vi "Steppers_and_Scanners_control_5_24.vi"(1 "ANC300 address":refnum<visa-resource-name>="COM8") -> (18 "Serial":string="ANC300B-C-2133-4009033")   [LabVIEW 2022 SP3]
panel:
  in  "wait time (ms)":u32=1
  out "2: Voltage Reading":dbl format="%#_13g"
  out "1: Voltage Reading":dbl format="%#_13g"
  in  "Set/Read":bool=TRUE
  in  "Stepper 4":bool
  in  "4: ms to wait":u32=1
  in  "4: number of steps":i32=1
  in  "4: stepping direction":bool=TRUE
  in  "4: AC Voltage":dbl=1.0 min=0.0 format="%.1g"
  in  "4: AC frequency":dbl=10.0 min=0.0 format="%.1f"
  in  "Stepper 3":bool
  in  "3: ms to wait":u32=1
  in  "3: number of steps":i32=1
  in  "3: stepping direction":bool=TRUE
  in  "3: AC Voltage":dbl=1.0 min=0.0 format="%.1g"
  in  "3: AC frequency":dbl=10.0 min=0.0 format="%.1f"
  in  "2: ms to wait":u32=1
  in  "2: Offset Voltage":dbl min=0.0 format="%.1g"
  in  "1: ms to wait":u32=1
  in  "1: Offset Voltage":dbl min=0.0 format="%.1g"
  # "Scanner 1"
  # "Scanner 2"
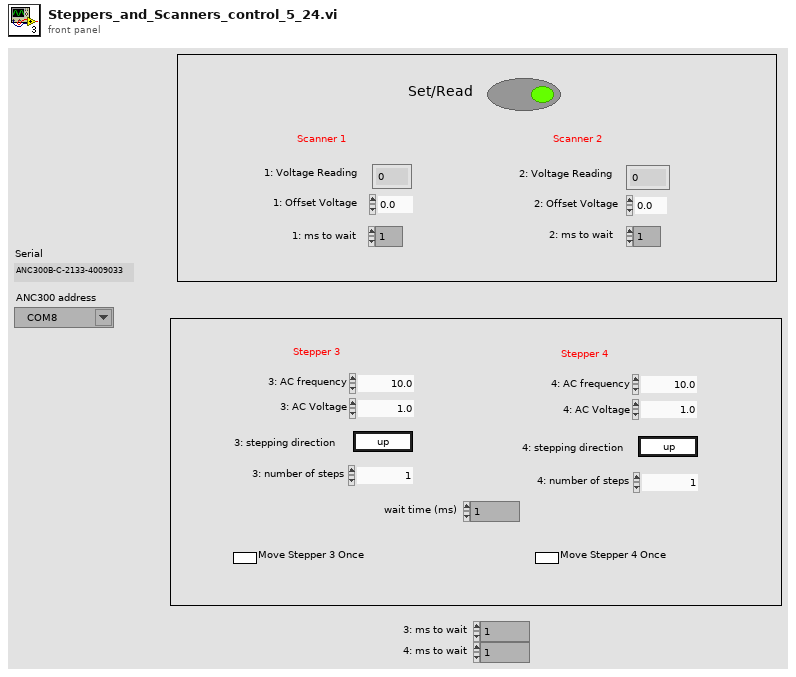
[diagram p1: front panel]
types:
  T1 = cluster{"error ":bool, "error number":i32, "error code":string}
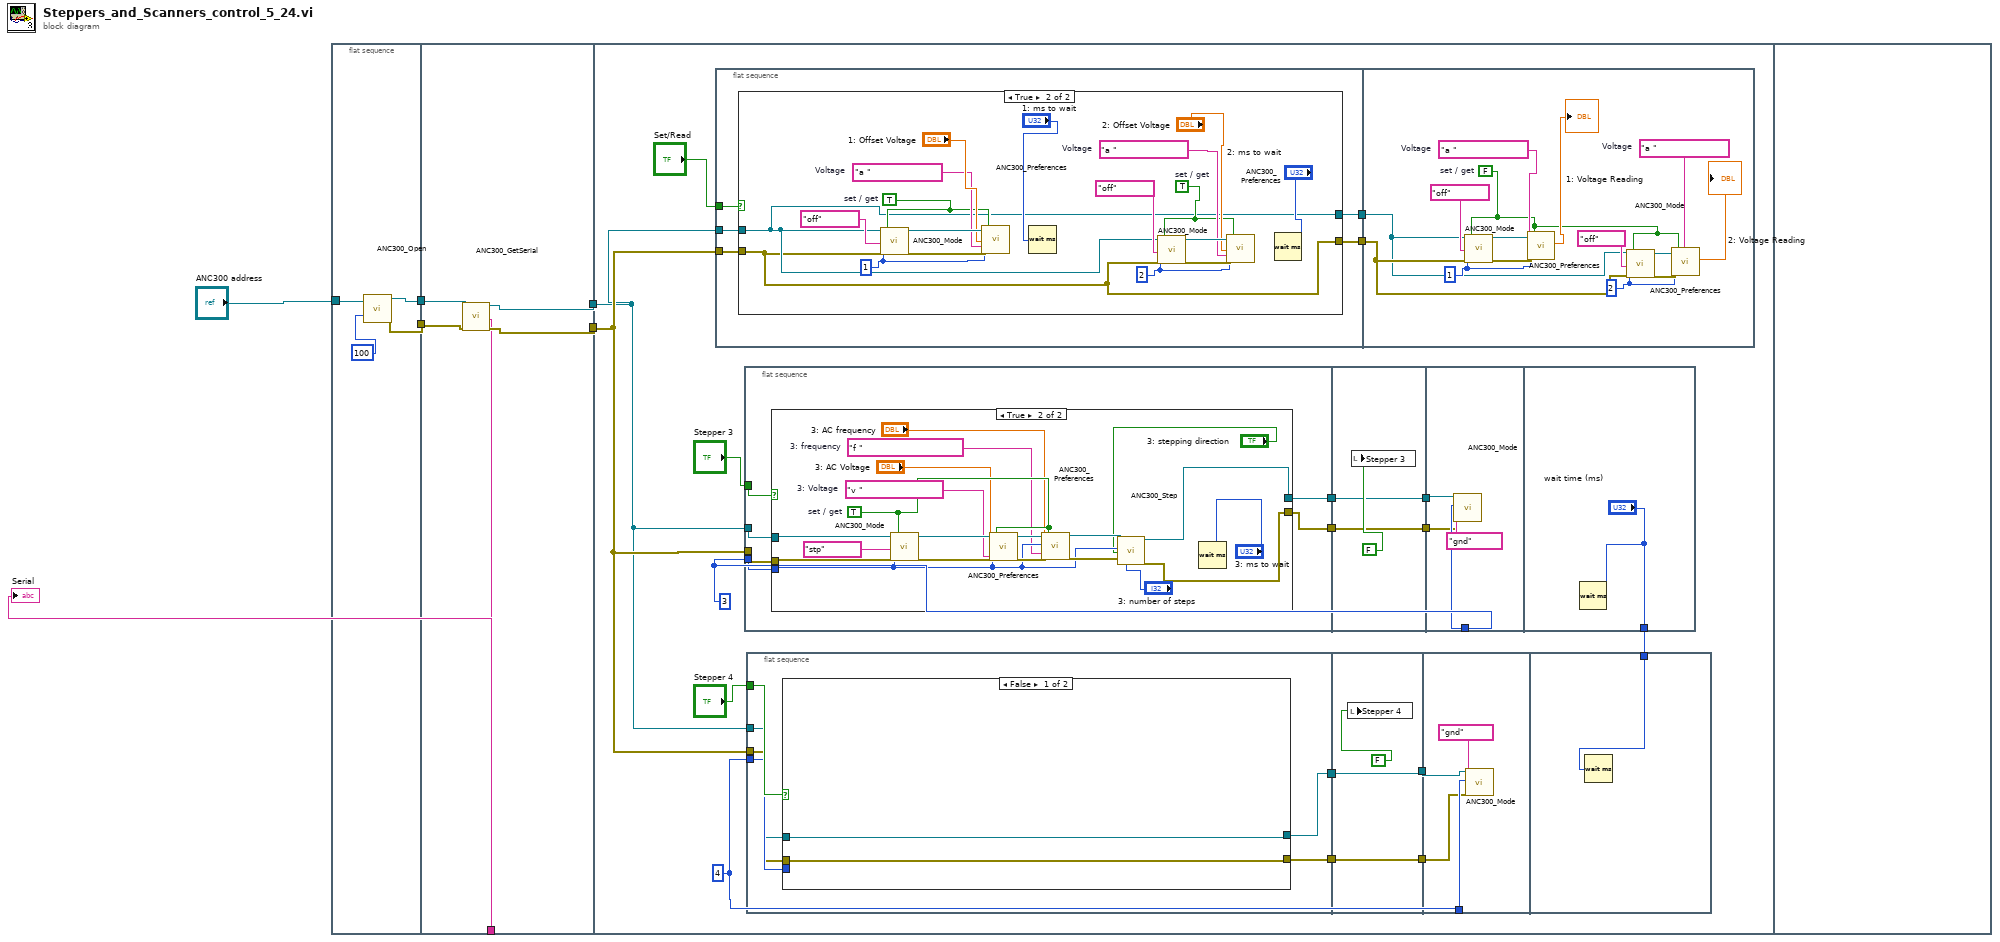
[diagram p0: block diagram]
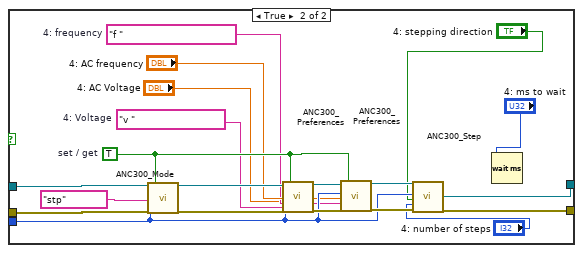
[diagram p4: hidden frame]
diagram:
  n1 = flat-sequence {
    tunnel: "ANC300 address" -> [w9]
    tunnel: [w10] -> w6
    tunnel: [w8] -> w5
    tunnel: w6 -> [w15]
    tunnel: w5 -> [w14]
    tunnel: [w13] -> w4
    tunnel: [w12] -> w3
    tunnel: [w11] -> w2
    tunnel: w4 -> [w30]
    tunnel: w3 -> [w31]
    frame #0 {
      n2 = call "ANC300_Open.vi"("ANC300 Communication Port In"=w9, "milliseconds to wait"=u32 100 ("millisecond timer value")) -> ("ANC300 Communication Port Out"=w10:refnum<visa-resource-name>, "error out"=w8:T1)  [unwired: 13 in, 3 out]
    }
    frame #1 {
      n3 = call "ANC300_GetSerial.vi"("ANC300 Communication Port In"=w15, "error in"=w14) -> ("ANC300 Communication Port Out"=w13:refnum<visa-resource-name>, "Serial"=w11:string, "error out"=w12:T1)  [unwired: 10 in, 5 out]
    }
    frame #2 {
      w29 = 3
      w32 = 4
      n4 = flat-sequence {
        tunnel: w31 -> [w38]
        tunnel: w30 -> [w37]
        tunnel: "Set/Read" -> [w36]
        tunnel: [w35] -> w22
        tunnel: [w34] -> w21
        tunnel: w22 -> [w62]
        tunnel: w21 -> [w63]
        frame #0 {
          n5 = case shown="True" w36 {
            tunnel: w38 -> [w39 w41]
            tunnel: w37 -> [w40 w42]
            tunnel: [w40 w42] -> w35
            tunnel: [w39 w41] -> w34
            frame False {
            }
            frame True {
              w43 = 2
              w44 = 1
              w45 = TRUE  # set / get
              w48 = "a "  # Voltage
              w52 = TRUE  # set / get
              w55 = "a "  # Voltage
              n6 = call "ANC300_Mode.vi"("ANC300 Communication Port In"=w42, "Axis"=w44, "axis mode in"="off", "error in"=w41, "set / get"=w52) -> ("ANC300 Communication Port Out"=w58:refnum<visa-resource-name>, "error out"=w57:T1)  [unwired: 8 in, 5 out]
              n7 = call "ANC300_Preferences.vi"("ANC300 Communication Port In"=w58, "Axis"=w44, "value in"="1: Offset Voltage", "parameter"=w55, "error in"=w57, "set / get"=w52) -> ()  [unwired: 6 in, 8 out]
              n8 = Wait (ms)(milliseconds to wait="1: ms to wait") -> ()  [unwired: 1 out]
              n9 = call "ANC300_Mode.vi"("ANC300 Communication Port In"=w42, "Axis"=w43, "axis mode in"="off", "error in"=w41, "set / get"=w45) -> ("ANC300 Communication Port Out"=w51:refnum<visa-resource-name>, "error out"=w50:T1)  [unwired: 8 in, 5 out]
              n10 = call "ANC300_Preferences.vi"("ANC300 Communication Port In"=w51, "Axis"=w43, "value in"="2: Offset Voltage", "parameter"=w48, "error in"=w50, "set / get"=w45) -> ()  [unwired: 6 in, 8 out]
              n11 = Wait (ms)(milliseconds to wait="2: ms to wait") -> ()  [unwired: 1 out]
            }
          }
        }
        frame #1 {
          w64 = 2
          w65 = 1
          w67 = "a "  # Voltage
          w59 = FALSE  # set / get
          w71 = "a "  # Voltage
          n12 = call "ANC300_Mode.vi"("ANC300 Communication Port In"=w62, "Axis"=w65, "axis mode in"="off", "error in"=w63, "set / get"=w59) -> ("ANC300 Communication Port Out"=w73:refnum<visa-resource-name>, "error out"=w72:T1)  [unwired: 8 in, 5 out]
          n13 = call "ANC300_Preferences.vi"("ANC300 Communication Port In"=w73, "Axis"=w65, "parameter"=w71, "error in"=w72, "set / get"=w59) -> ("value out"=→"1: Voltage Reading":dbl)  [unwired: 7 in, 7 out]
          n14 = call "ANC300_Mode.vi"("ANC300 Communication Port In"=w62, "Axis"=w64, "axis mode in"="off", "error in"=w63, "set / get"=w59) -> ("ANC300 Communication Port Out"=w69:refnum<visa-resource-name>, "error out"=w68:T1)  [unwired: 8 in, 5 out]
          n15 = call "ANC300_Preferences.vi"("ANC300 Communication Port In"=w69, "Axis"=w64, "parameter"=w67, "error in"=w68, "set / get"=w59) -> ("value out"=→"2: Voltage Reading":dbl)  [unwired: 7 in, 7 out]
        }
      }
      n16 = flat-sequence {
        tunnel: "Stepper 3" -> [w79]
        tunnel: w29 -> [w78]
        tunnel: w30 -> [w77]
        tunnel: w31 -> [w76]
        tunnel: [w75] -> w24
        tunnel: [w74] -> w19
        tunnel: [w103] -> w25
        tunnel: w24 -> [w103]
        tunnel: [w102] -> w20
        tunnel: w19 -> [w102]
        tunnel: w29 -> [w107]
        tunnel: w25 -> [w106]
        tunnel: w20 -> [w105]
        tunnel: ["wait time (ms)"] -> w16
        frame #0 {
          n17 = case shown="True" w79 {
            tunnel: w77 -> [w81 w101]
            tunnel: w78 -> [_ w93]
            tunnel: w76 -> [w80 w98]
            tunnel: [w81 w92] -> w75
            tunnel: [w80 w82] -> w74
            frame False {
            }
            frame True {
              w84 = "v "  # 3: Voltage
              w86 = "f "  # 3: frequency
              w89 = TRUE  # set / get
              n18 = call "ANC300_Mode.vi"("ANC300 Communication Port In"=w101, "Axis"=w93, "axis mode in"="stp", "error in"=w98, "set / get"=w89) -> ("ANC300 Communication Port Out"=w100:refnum<visa-resource-name>, "error out"=w97:T1)  [unwired: 8 in, 5 out]
              n19 = call "ANC300_Preferences.vi"("ANC300 Communication Port In"=w100, "Axis"=w93, "value in"="3: AC Voltage", "parameter"=w84, "error in"=w97, "set / get"=w89) -> ("ANC300 Communication Port Out"=w95:refnum<visa-resource-name>, "error out"=w94:T1)  [unwired: 6 in, 6 out]
              n20 = call "ANC300_Preferences.vi"("ANC300 Communication Port In"=w95, "Axis"=w93, "value in"="3: AC frequency", "parameter"=w86, "error in"=w94, "set / get"=w89) -> ("ANC300 Communication Port Out"=w99:refnum<visa-resource-name>, "error out"=w96:T1)  [unwired: 6 in, 6 out]
              n21 = call "ANC300_Step.vi"("ANC300 Communication Port In"=w99, "Axis"=w93, "stepping direction"="3: stepping direction", "number of steps [0=cont.]"="3: number of steps", "error in"=w96) -> ("ANC300 Communication Port Out"=w92:refnum<visa-resource-name>, "error out"=w82:T1)  [unwired: 9 in, 4 out]
              n22 = Wait (ms)(milliseconds to wait="3: ms to wait") -> ()  [unwired: 1 out]
            }
          }
        }
        frame #1 {
          n23 = local write "Stepper 3"(FALSE) -> ()
        }
        frame #2 {
          n24 = call "ANC300_Mode.vi"("ANC300 Communication Port In"=w106, "Axis"=w107, "axis mode in"="gnd" ("3 Stepper x"), "error in"=w105) -> ()  [unwired: 9 in, 7 out]
        }
        frame #3 {
          n25 = Wait (ms)(milliseconds to wait="wait time (ms)") -> ()  [unwired: 1 out]
        }
      }
      n26 = flat-sequence {
        tunnel: "Stepper 4" -> [w115]
        tunnel: w32 -> [w114]
        tunnel: w30 -> [w113]
        tunnel: w31 -> [w112]
        tunnel: [w111] -> w26
        tunnel: [w110] -> w17
        tunnel: [w139] -> w27
        tunnel: w26 -> [w139]
        tunnel: [w138] -> w18
        tunnel: w17 -> [w138]
        tunnel: w32 -> [w143]
        tunnel: w27 -> [w142]
        tunnel: w18 -> [w141]
        tunnel: w16 -> [w145]
        frame #0 {
          n27 = case shown="False" w115 {
            tunnel: w113 -> [w117 w137]
            tunnel: w114 -> [_ w129]
            tunnel: w112 -> [w116 w134]
            tunnel: [w117 w128] -> w111
            tunnel: [w116 w118] -> w110
            frame False {
            }
            frame True {
              w123 = "v "  # 4: Voltage
              w121 = "f "  # 4: frequency
              w125 = TRUE  # set / get
              n28 = call "ANC300_Mode.vi"("ANC300 Communication Port In"=w137, "Axis"=w129, "axis mode in"="stp", "error in"=w134, "set / get"=w125) -> ("ANC300 Communication Port Out"=w136:refnum<visa-resource-name>, "error out"=w133:T1)  [unwired: 8 in, 5 out]
              n29 = call "ANC300_Preferences.vi"("ANC300 Communication Port In"=w136, "Axis"=w129, "value in"="4: AC Voltage", "parameter"=w123, "error in"=w133, "set / get"=w125) -> ("ANC300 Communication Port Out"=w131:refnum<visa-resource-name>, "error out"=w130:T1)  [unwired: 6 in, 6 out]
              n30 = call "ANC300_Preferences.vi"("ANC300 Communication Port In"=w131, "Axis"=w129, "value in"="4: AC frequency", "parameter"=w121, "error in"=w130, "set / get"=w125) -> ("ANC300 Communication Port Out"=w135:refnum<visa-resource-name>, "error out"=w132:T1)  [unwired: 6 in, 6 out]
              n31 = call "ANC300_Step.vi"("ANC300 Communication Port In"=w135, "Axis"=w129, "stepping direction"="4: stepping direction", "number of steps [0=cont.]"="4: number of steps", "error in"=w132) -> ("ANC300 Communication Port Out"=w128:refnum<visa-resource-name>, "error out"=w118:T1)  [unwired: 9 in, 4 out]
              n32 = Wait (ms)(milliseconds to wait="4: ms to wait") -> ()  [unwired: 1 out]
            }
          }
        }
        frame #1 {
          n33 = local write "Stepper 4"(FALSE) -> ()
        }
        frame #2 {
          n34 = call "ANC300_Mode.vi"("ANC300 Communication Port In"=w142, "Axis"=w143, "axis mode in"="gnd" ("3 Stepper x"), "error in"=w141) -> ()  [unwired: 9 in, 7 out]
        }
        frame #3 {
          n35 = Wait (ms)(milliseconds to wait=w145) -> ()  [unwired: 1 out]
        }
      }
    }
    frame #3 {
    }
  }
  "Serial" <- w2
